vi "Processing Data.vi"(6 "Message":string, 7 "Total Iter":i32, 8 "error in (no error)":errorcluster, 10 "Current Iter":i32) -> (0 "error out":errorcluster, 2 "Cancel?":bool)   [LabVIEW 2017]
panel:
  in  "Cancel":bool
  out "Progress Bar":u8(slide) caption="Processing data..." max=1 step=1 scale=0.0..100.0
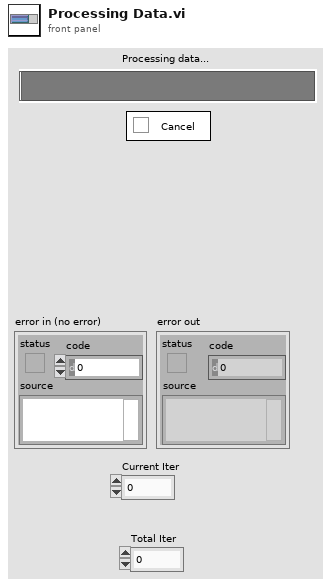
[diagram p1: front panel]
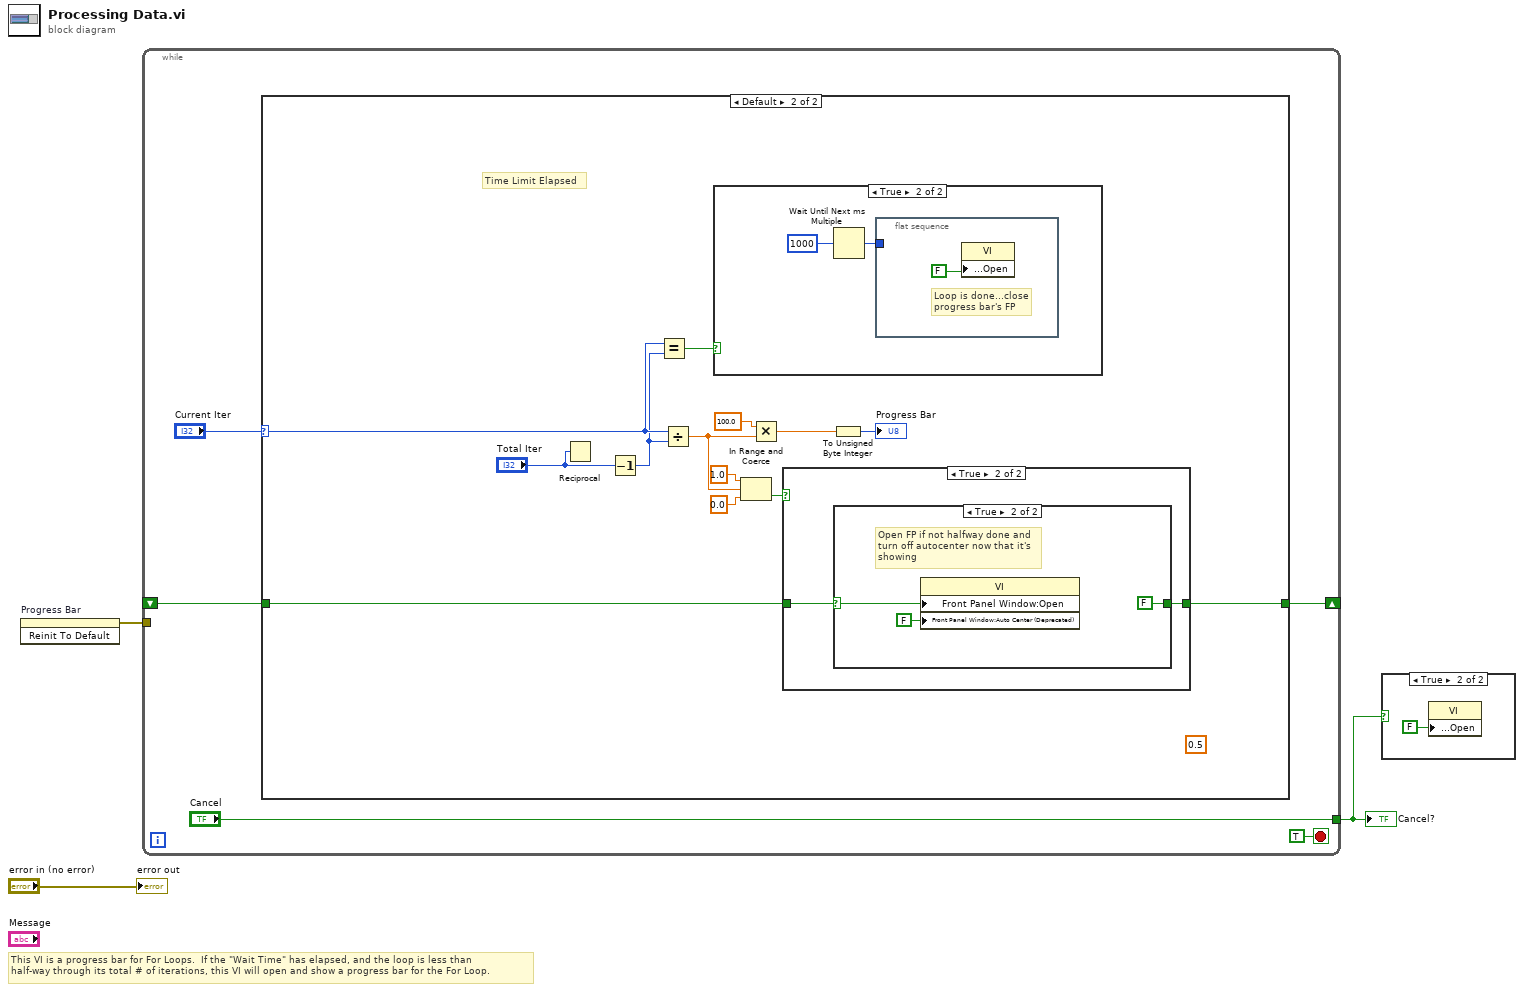
[diagram p0: block diagram]
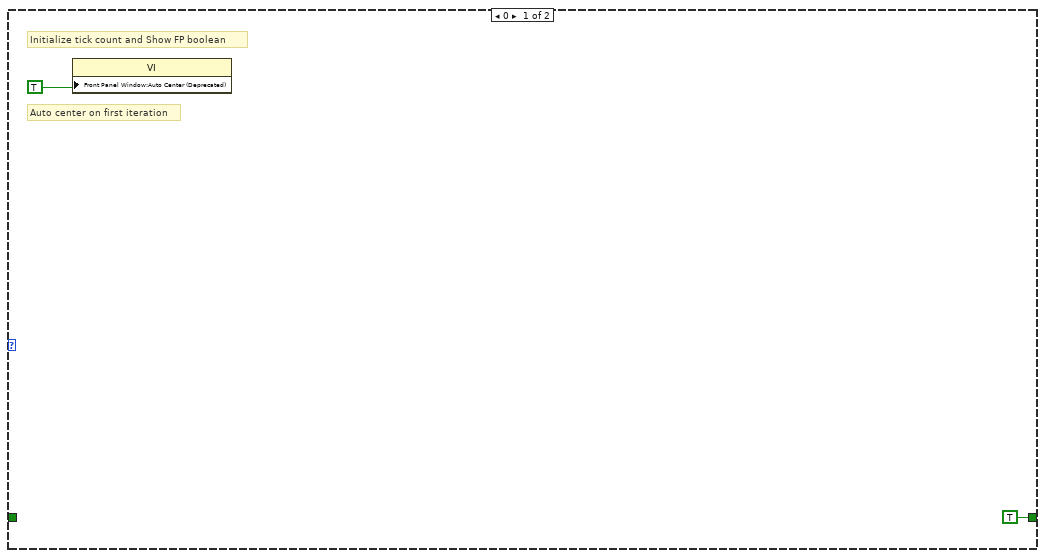
[diagram p3: hidden frame]
diagram:
  # "This VI is a progress bar for For Loops.  If the \"Wait Time\" has elapsed, and the loop is less than\nhalf-way through its total # of iterations, this VI will open and show a progress bar for the For Loop."
  n1 = invoke on="Progress Bar" class="Slide (strict)" method="Reinit To Default"() -> (error out=w2:errorcluster)  [unwired: 3 in, 2 out]
  n2 = while {
    shift-right: [w5] -> _
    shift-left: _ -> [w6]
    tunnel: w2 -> [_]
    tunnel: ["Cancel"] -> w1
    stop <- TRUE stop-if-true
    n3 = case shown="Default" "Current Iter" {
      selector: "Current Iter" -> [_ w23]
      tunnel: w6 -> [_ w22]
      tunnel: [TRUE w21] -> w5
      frame 0 {
        # "Auto center on first iteration"
        # "Initialize tick count and Show FP boolean"
        n4 = property class="VI"("Front Panel Window:Auto Center (Deprecated)"=TRUE ("Front Panel Window:Auto Center")) -> ()  [unwired: 2 in, 2 out]
      }
      frame Default {
        (unwired) 0.5 ("y")
        # "Time Limit Elapsed"
        n5 = Reciprocal(x="Total Iter") -> ()  [unwired: 1 out]
        n6 = Decrement(x="Total Iter") -> (x-1=w18:i32)
        n7 = Equal?(x=w23, y=w18) -> (x = y?=w20:bool)
        n8 = Divide(x=w23, y=w18) -> (x/y=w12:dbl)
        n9 = case shown="True" w20 {
          frame False {
            # "Loop is not done"
          }
          frame True {
            n10 = Wait Until Next ms Multiple(millisecond multiple=u32 1000) -> (millisecond timer value=w24:u32)
            n11 = flat-sequence {
              tunnel: w24 -> [_]
              frame #0 {
                # "Loop is done...close progress bar's FP"
                n12 = property class="VI"("Front Panel Window:Open"=FALSE) -> ()  [unwired: 2 in, 2 out]
              }
            }
          }
        }
        n13 = In Range and Coerce(upper limit=1.0, x=w12, lower limit=0.0) -> (In Range?=w19:bool)  [unwired: 1 out]
        n14 = Multiply(x=100.0, y=w12) -> (x*y=w14:dbl)
        n15 = case shown="True" w19 {
          tunnel: w22 -> [w27 w29]
          tunnel: [w27 w28] -> w21
          frame False {
            # "Progress is over halfway done...just wait it out with no progress bar"
          }
          frame True {
            n16 = case shown="True" w29 {
              selector: w29 -> [w30 w33]
              tunnel: [w30 FALSE] -> w28
              frame False {
                # "FP has already been opened"
              }
              frame True {
                # "Open FP if not halfway done and turn off autocenter now that it's showing"
                n17 = property class="VI"("Front Panel Window:Open"=w33, "Front Panel Window:Auto Center (Deprecated)"=FALSE) -> ()  [unwired: 2 in, 2 out]
              }
            }
          }
        }
        n18 = To Unsigned Byte Integer(number=w14) -> (unsigned 8bit integer=→"Progress Bar":u8)
      }
    }
  }
  "Cancel?" <- w1
  n19 = case shown="True" w1 {
    frame False {
    }
    frame True {
      n20 = property class="VI"("Front Panel Window:Open"=FALSE) -> ()  [unwired: 2 in, 2 out]
    }
  }
  "error out" <- "error in (no error)"
